vi "计算MES_PSNR值.vi"(0 "ori":dbl[][](array[numeric]), 1 "rec":dbl[][](array[numeric])) -> (3 "MSE":dbl, 4 "PSNR":dbl, 5 "SNR":dbl)   [LabVIEW 2018]
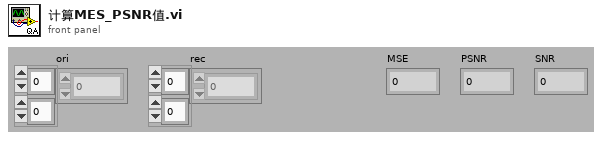
[diagram p1: front panel]
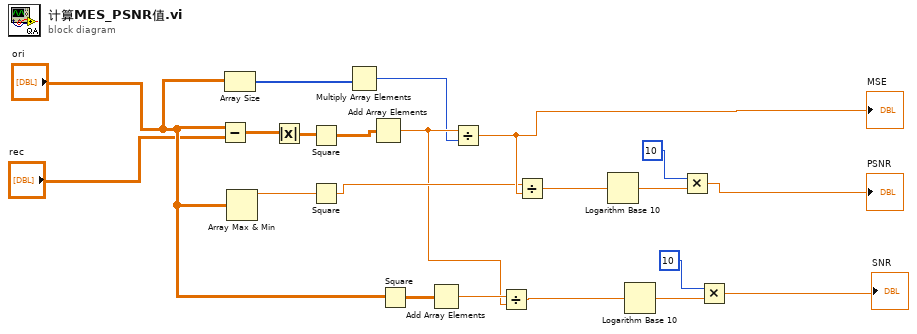
[diagram p0: block diagram]
diagram:
  n1 = Subtract(x="ori", y="rec") -> (x-y=w3:dbl[][])
  n2 = Array Size ("数组大小")(array="ori") -> (size(s)=w2:i32[])
  n3 = Array Max & Min(array="ori") -> (max value=w17:dbl)  [unwired: 3 out]
  n4 = Absolute Value(x=w3) -> (abs(x)=w19:dbl[][])
  n5 = Square(x=w19) -> (x^2=w20:dbl[][])
  n6 = Square(x=w17) -> (x^2=w18:dbl)
  n7 = Multiply Array Elements(1:w2) -> (0:w1:i32)
  n8 = Add Array Elements(numeric array=w20) -> (sum=w10:dbl)
  n9 = Square(x="ori") -> (x^2=w12:dbl[][])
  n10 = Add Array Elements(numeric array=w12) -> (sum=w11:dbl)
  n11 = Divide(x=w10, y=w1) -> (x/y=w21:dbl)
  "MSE" <- w21
  n12 = Divide(x=w11, y=w10) -> (x/y=w7:dbl)
  n13 = Divide(x=w18, y=w21) -> (x/y=w16:dbl)
  n14 = Logarithm Base 10(1:w16) -> (0:w15:dbl)
  n15 = Logarithm Base 10(1:w7) -> (0:w8:dbl)
  n16 = Multiply(x=u8 10, y=w15) -> (x*y=→"PSNR":dbl)
  n17 = Multiply(x=u8 10, y=w8) -> (x*y=→"SNR":dbl)
